vi "Thermotest.vi"() -> ()   [LabVIEW 2020]
panel:
  out "TC6":dbl
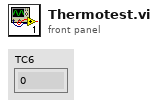
[diagram p1: front panel]
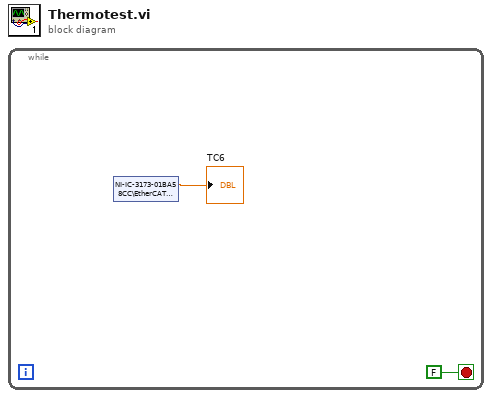
[diagram p0: block diagram]
diagram:
  n1 = while {
    stop <- FALSE stop-if-true
    n2 = shared-variable "NI-IC-3173-01BA58CC\\EtherCAT Master\\Device\\Mod3\\TC7"() -> (→"TC6":dbl)  [unwired: 1 in, 1 out]
  }
